vi "Start test.vi"(8 "error in":errorcluster, 9 "Set voltage":i32=4500, 10 "Set time":i32=60, 11 "Megger cluster in":T1={"Read data"={"Firmware version"="", "Model number"="", "Serial number"=0, "Ramp rate"=0.0, "Test Voltage"=0.0, "Test duration"=0.0, "Test stop watch"=0.0, "measured Current (nA)"=0.0, "calculated Resistance"=0.0, "Test Mode"=enum."Insulation resistance (IR)", "Test status"=enum."Waiting to start test"}, "Connected?"=FALSE, "Device status array"=[]}) -> (0 "error out":errorcluster, 3 "Megger cluster out":T1={"Read data"={"Firmware version"="", "Model number"="", "Serial number"=0, "Ramp rate"=0.0, "Test Voltage"=0.0, "Test duration"=0.0, "Test stop watch"=0.0, "measured Current (nA)"=0.0, "calculated Resistance"=0.0, "Test Mode"=enum."Insulation resistance (IR)", "Test status"=enum."Waiting to start test"}, "Connected?"=FALSE, "Device status array"=[]})   [LabVIEW 2014]
doc: "This function is used to start a timed insulation resistance test on the device. A test voltage and test duration will need to be supplied. Note: This VI will take 5 seconds to set test up and will be locked out during this time."
uses:
  Private/Controls/Megger cluster.ctl
  Private/Controls/Global Megger.vi
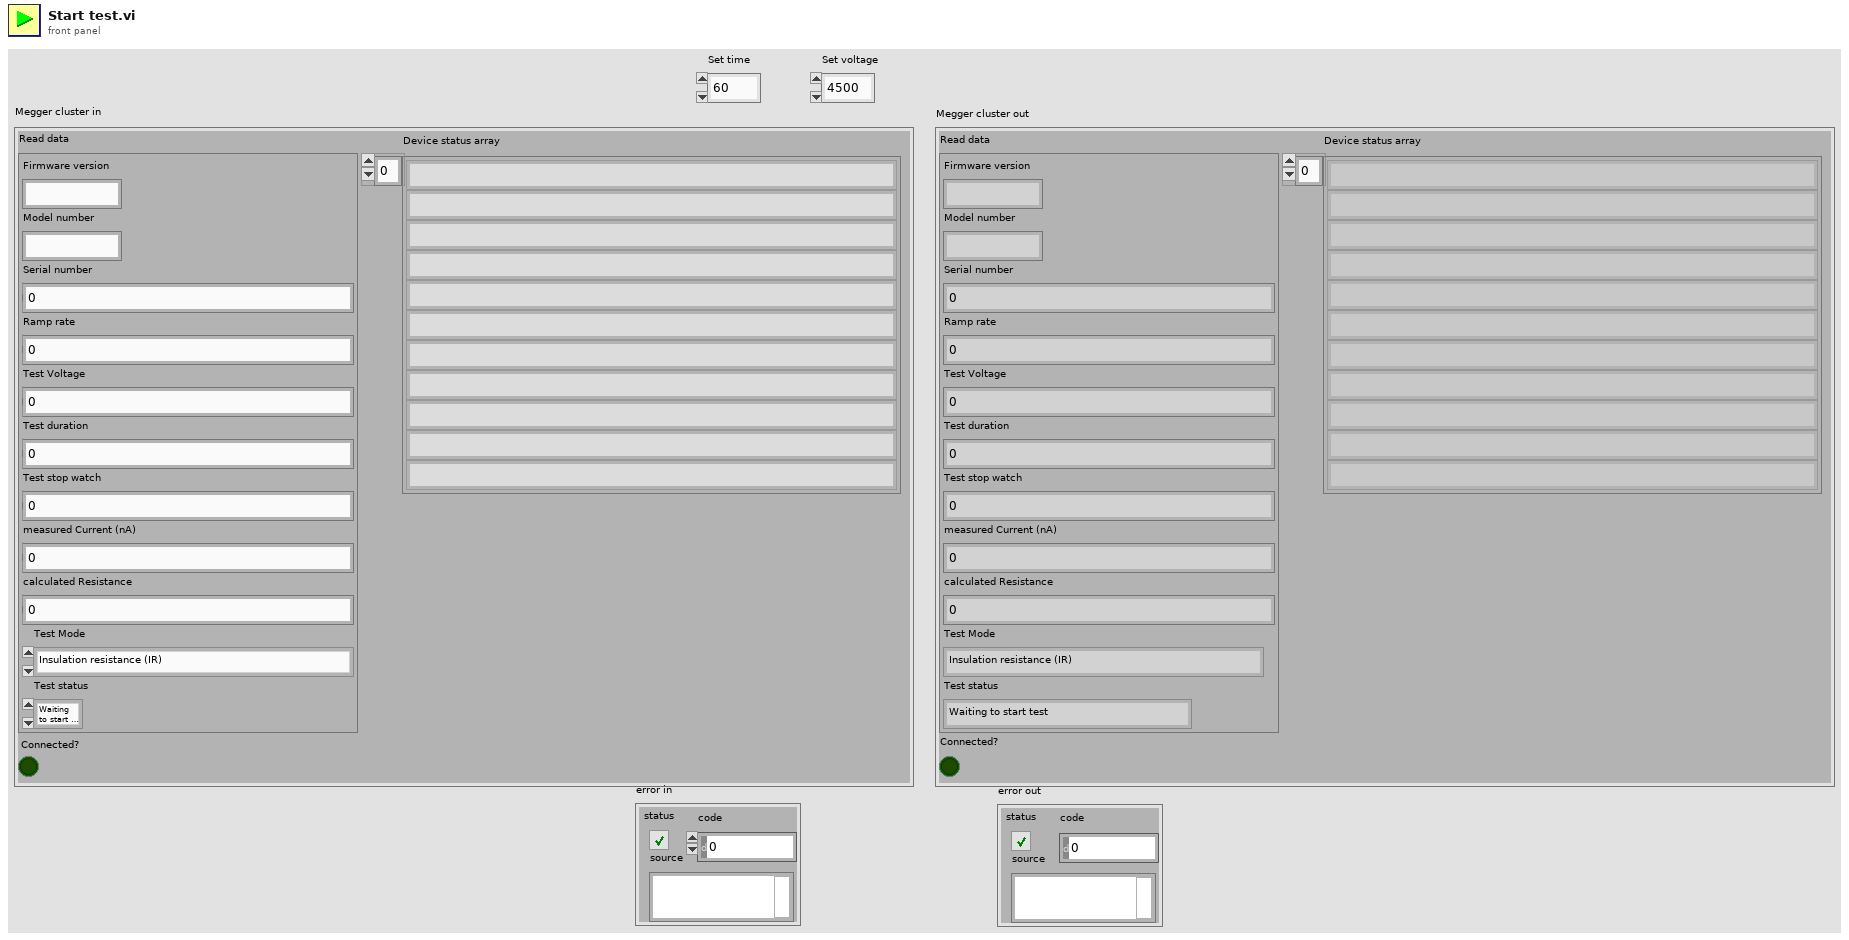
[diagram p1: front panel]
types:
  T1 = typedef "Megger cluster.ctl" = cluster{"Read data":cluster{"Firmware version":string, "Model number":string, "Serial number":i32, "Ramp rate":dbl, "Test Voltage":dbl, "Test duration":sgl, "Test stop watch":sgl, "measured Current (nA)":dbl, "calculated Resistance":dbl, "Test Mode":enum16{"N/A", "Insulation resistance (IR)", "Timed Insulation resistance (IR(t))", "Diaelectric Absorption Ratio (DAR)", "Polarisation Index (PI)", "Diaelectric Dishcharge (DD)", "Step voltage (SV)", "Ramp test (Ramp)"}, "Test status":enum16{"Waiting to start test", "Unable to start test", "Test progressing normally", "Performing post test measurements", "Test has ended normally", "Test has been aborted"}}, "Connected?":bool, "Device status array":string[]}
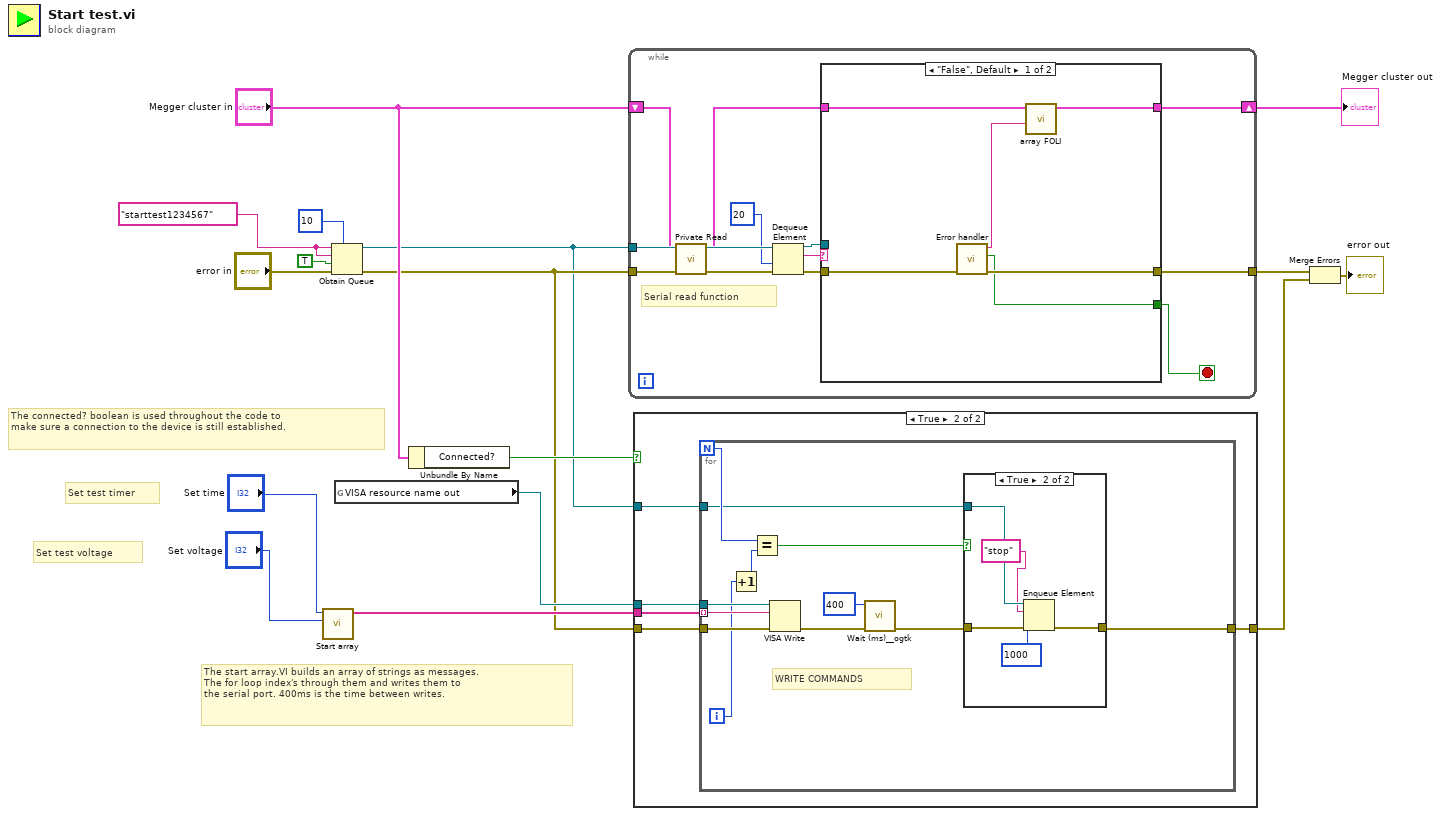
[diagram p0: block diagram]
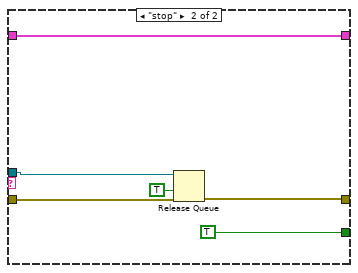
[diagram p2: hidden frame]
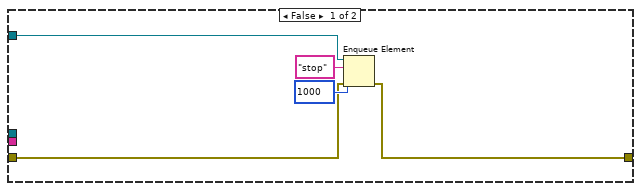
[diagram p3: hidden frame]
diagram:
  w6 = "starttest1234567" ("name (unnamed)")
  # "The start array.VI builds an array of strings as messages.\nThe for loop index's through them and writes them to \nthe serial port. 400ms is the time between writes."
  # "The connected? boolean is used throughout the code to\nmake sure a connection to the device is still established."
  # "Set test timer"
  # "Set test voltage"
  n1 = call "Start array.vi"("Set voltage"="Set voltage", "Set time"="Set time") -> ("Start array"=w14:string[])  [unwired: 9 in]
  n2 = Obtain Queue(max queue size (-1, unlimited)=10, name (unnamed)=w6, element data type=w6, create if not found? (T)=TRUE, error in (no error)="error in") -> (queue out=w3:refnum<queue>, error out=w4:errorcluster)  [unwired: 1 out]
  n3 = global read "Global Megger.vi" "VISA resource name out"() -> (w13:refnum<visa-resource-name>)
  n4 = Unbundle By Name("Megger cluster in") -> ("Connected?"=w9:bool)
  n5 = while {
    tunnel: w4 -> [w24]
    tunnel: w3 -> [w28]
    tunnel: [w20] -> w2
    shift-right: [w17] -> w1
    shift-left: "Megger cluster in" -> [w23]
    stop <- w21 stop-if-true
    # "Serial read function"
    n6 = call "Private Read.vi"("error in"=w24, "Megger cluster in"=w23) -> ("error out"=w25:errorcluster, "Megger cluster out"=w22:T1)  [unwired: 7 in, 1 out]
    n7 = Dequeue Element(queue=w28, timeout in ms (-1)=20, error in (no error)=w25) -> (queue out=w18:refnum<queue>, element=w27:string, error out=w19:errorcluster)  [unwired: 1 out]
    n8 = case shown="\"False\", Default" w27 {
      tunnel: w22 -> [w31 w39]
      tunnel: [w32 TRUE] -> w21
      tunnel: [w30 w39] -> w17
      tunnel: [w33 w37] -> w20
      tunnel: w19 -> [w34 w38]
      tunnel: w18 -> [_ w36]
      frame "False", Default {
        n9 = call "Error handler.vi"("error in"=w34) -> ("error out"=w33:errorcluster, "status"=w32:bool, "Status string"=w29:string)  [unwired: 8 in]
        n10 = call "array FOLI.vi"("status string"=w29, "Megger cluster in"=w31) -> ("Megger cluster out"=w30:T1)  [unwired: 9 in]
      }
      frame "stop" {
        n11 = Release Queue(queue=w36, force destroy? (F)=TRUE, error in (no error)=w38) -> (error out=w37:errorcluster)  [unwired: 2 out]
      }
    }
  }
  "Megger cluster out" <- w1
  n12 = case shown="True" w9 {
    tunnel: w14 -> [_ w50]
    tunnel: w4 -> [w42 w49]
    tunnel: w13 -> [_ w48]
    tunnel: [w41 w47] -> w11
    tunnel: w3 -> [w43 w46]
    frame False {
      n13 = Enqueue Element(queue=w43, element="stop", timeout in ms (-1)=1000, error in (no error)=w42) -> (error out=w41:errorcluster)  [unwired: 2 out]
    }
    frame True {
      n14 = for {
        N -> [w57]
        tunnel: w50 -> [w62] mode=indexing
        tunnel: w49 -> [w61]
        tunnel: w48 -> [w60]
        tunnel: [w53] -> w47
        tunnel: w46 -> [w55]
        i -> [w52]
        # "WRITE COMMANDS"
        n15 = Increment(x=w52) -> (x+1=w51:i32)
        n16 = Equal?(x=w57, y=w51) -> (x = y?=w56:bool)
        n17 = VISA Write(VISA resource name=w60, write buffer=w62, error in (no error)=w61) -> (error out=w59:errorcluster)  [unwired: 2 out]
        n18 = call <userlib>:"Wait (ms)__ogtk.vi"("error in (no error)"=w59, "milliseconds to wait"=u32 400) -> ("error out"=w54:errorcluster)  [unwired: 8 in, 1 out]
        n19 = case shown="True" w56 {
          tunnel: w55 -> [_ w68]
          tunnel: w54 -> [w63 w67]
          tunnel: [w63 w66] -> w53
          frame False {
          }
          frame True {
            n20 = Enqueue Element(queue=w68, element="stop", timeout in ms (-1)=1000, error in (no error)=w67) -> (error out=w66:errorcluster)  [unwired: 2 out]
          }
        }
      }
    }
  }
  n21 = Merge Errors(w2, w11) -> (→"error out":errorcluster)
